vi "ResultGame.vi"(10 "EndData":T1, 11 "MainData":T3={"Image"={"image type"=0, "image depth"=32, "image"=array[640000 elements], "mask"=array[20000 elements], "colors"=[], "Rectangle"={"left"=0, "top"=0, "right"=400, "bottom"=400}}, " TmpImage"={"image type"=0, "image depth"=32, "image"=array[640000 elements], "mask"=array[20000 elements], "colors"=[], "Rectangle"={"left"=0, "top"=0, "right"=400, "bottom"=400}}, "BGColor"=15256322, "FGColor"=13283586, "DRColor"=13283586, "Picture"=bytes[500030], "Queue "=refnum, "EndGameEvent"=refnum, "AnalizeMove"=FALSE}) -> (3 "Result info":string)   [LabVIEW 2020]
doc: "Prepare description with game result."
uses:
  typeDef/MainDataCluster.ctl
  <vilib>/picture/picture.llb/imagedata.ctl
  typeDef/StateMachineEnum.ctl
  typeDef/EventData.ctl
  typeDef/EndType.ctl
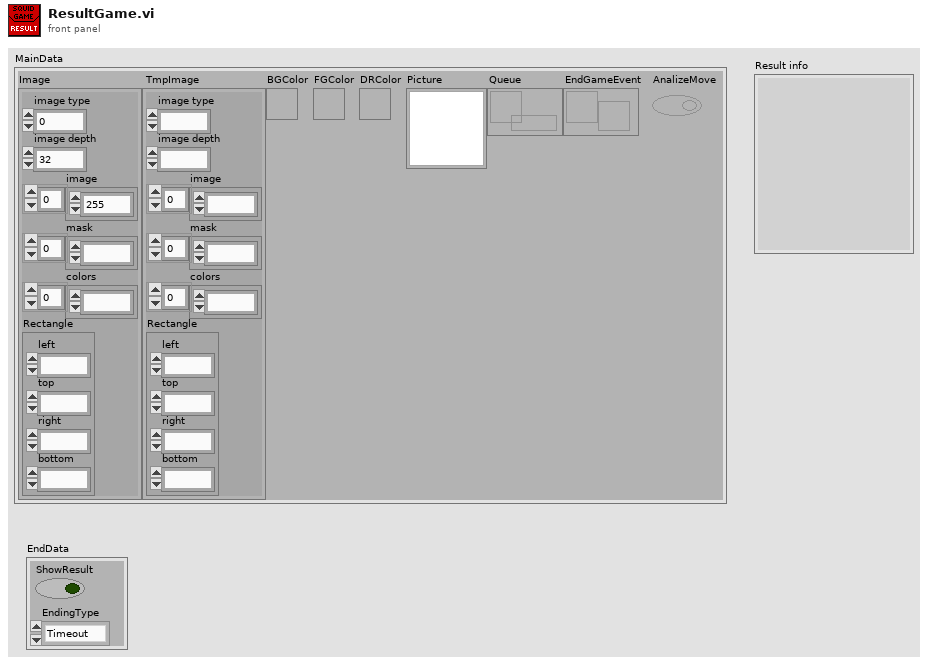
[diagram p1: front panel]
types:
  T1 = typedef "EventData.ctl" = cluster{"ShowResult":bool, "EndingType":T2}
  T2 = typedef "EndType.ctl" = enum16{"Timeout", "MouseUp", "OutOfLine", "CloseLine", "UserEnd"}
  T3 = typedef "MainDataCluster.ctl" = cluster{"Image":T4, " TmpImage":T4, "BGColor":u32, "FGColor":u32, "DRColor":u32, "Picture":picture, "Queue ":refnum<queue>, "EndGameEvent":refnum<user-event>, "AnalizeMove":bool}
  T4 = typedef "imagedata.ctl" = cluster{"image type":i32, "image depth":i32, "image":u8[], "mask":u8[], "colors":u32[], "Rectangle":cluster{"left":i16, "top":i16, "right":i16, "bottom":i16}}
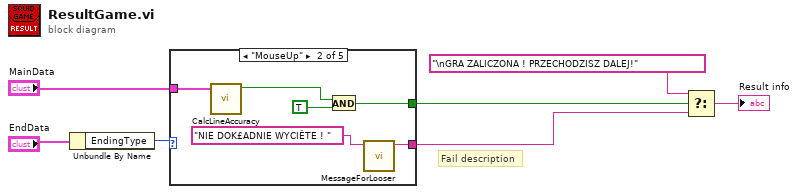
[diagram p0: block diagram]
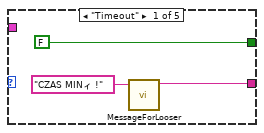
[diagram p2: hidden frame]
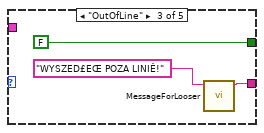
[diagram p3: hidden frame]
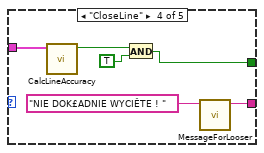
[diagram p4: hidden frame]
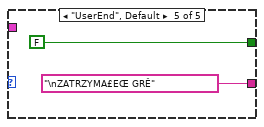
[diagram p5: hidden frame]
diagram:
  # "Fail description"
  n1 = Unbundle By Name("EndData") -> ("EndingType"=w5:T2)
  n2 = case shown="\"MouseUp\"" w5 {
    tunnel: [FALSE w15 FALSE w24 FALSE] -> w3
    tunnel: [w8 w13 w17 w22 "\nZATRZYMA£EŒ GRÊ" ("String out")] -> w2
    tunnel: "MainData" -> [_ w12 _ w21 _]
    frame "Timeout" {
      n3 = call "MessageForLooser.vi"("String in"="CZAS MINィ !") -> ("String out"=w8:string)  [unwired: 10 in]
    }
    frame "MouseUp" {
      n4 = call "CalcLineAccuracy.vi"("MainData"=w12) -> ("Good ?"=w11:bool)  [unwired: 10 in]
      n5 = And(x=w11, y=TRUE) -> (x .and. y?=w15:bool)
      n6 = call "MessageForLooser.vi"("String in"="NIE DOK£ADNIE WYCIÊTE ! ") -> ("String out"=w13:string)  [unwired: 10 in]
    }
    frame "OutOfLine" {
      n7 = call "MessageForLooser.vi"("String in"="WYSZED£EŒ POZA LINIÊ!") -> ("String out"=w17:string)  [unwired: 10 in]
    }
    frame "CloseLine" {
      n8 = call "CalcLineAccuracy.vi"("MainData"=w21) -> ("Good ?"=w20:bool)  [unwired: 10 in]
      n9 = And(x=w20, y=TRUE) -> (x .and. y?=w24:bool)
      n10 = call "MessageForLooser.vi"("String in"="NIE DOK£ADNIE WYCIÊTE ! ") -> ("String out"=w22:string)  [unwired: 10 in]
    }
    frame "UserEnd", Default {
    }
  }
  n11 = Select(t="\nGRA ZALICZONA ! PRZECHODZISZ DALEJ!" ("T button name (\"OK\")"), s=w3, f=w2) -> (s? t:f=→"Result info":string)
